vi "Tag Names.vi"(11 "Process Name":string) -> (2 "SC Tags":T1, 4 "All Boolean Tags":string[](array[string]), 5 "All  Numeric Tags":string[](array[string]))   [LabVIEW 2018, in "Sonicator Module.lvlib" / "Sonicator Module Engine.lvlib"]
uses:
  Sonicator Module Engine.lvlib
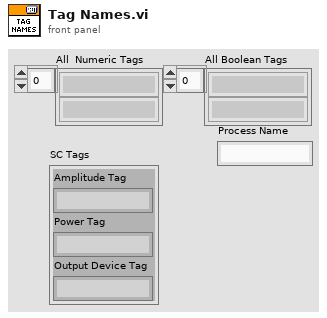
[diagram p1: front panel]
types:
  T1 = cluster{"Amplitude Tag":string, "Power Tag":string, "Output Device Tag":string}
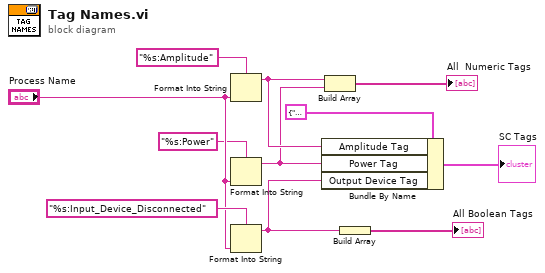
[diagram p0: block diagram]
diagram:
  n1 = Format Into String(format string="%s:Amplitude", "Process Name") -> (resulting string=w7:string)  [unwired: 2 in, 1 out]
  n2 = Format Into String(format string="%s:Power", "Process Name") -> (resulting string=w1:string)  [unwired: 2 in, 1 out]
  n3 = Format Into String(format string="%s:Input_Device_Disconnected", "Process Name") -> (resulting string=w4:string)  [unwired: 2 in, 1 out]
  n4 = Bundle By Name(cluster=T1 {"Amplitude Tag"="", "Power Tag"="", "Output Device Tag"=""} ("SC Tags"), "Amplitude Tag"=w7, "Power Tag"=w1, "Output Device Tag"=w4) -> (→"SC Tags":T1)
  n5 = Build Array(w7, w1) -> (→"All  Numeric Tags":string[])
  n6 = Build Array(w4) -> (→"All Boolean Tags":string[])
